vi "Icai 105 - Simultry4.vi"() -> ()   [LabVIEW 2010]
uses:
  <vilib>/Utility/error.llb/DialogType.ctl
  <vilib>/DAQmx/write.llb/DAQmx Write (Analog DBL 1Chan 1Samp).vi
  <vilib>/DAQmx/write.llb/DAQmx Write (Analog Wfm 1Chan NSamp).vi
  <vilib>/DAQmx/create/channels.llb/DAQmx Create Channel (AO-Voltage-Basic).vi
  <vilib>/daqmx/miscellaneous.llb/DAQmx Fill In Error Info.vi
  <vilib>/Waveform/WDTOps.llb/WDT Append Waveforms DBL.vi
  <vilib>/measure/NI_MABase.lvlib
  Program Files/National Instruments/LabVIEW 2010/resource/objmgr/daqmx.rc
panel:
  in  "Rising Logic Output Chan":tag="Dev1/ao2"
  in  "Modulation Duration samples / 2":i32=150000
  out "Multiplier to arrive at Modulation # of samples":dbl=297.555285
  in  "Samples (1Ms/s)":i32=700000
  out "Name":refnum<k21>
  out "number of samples written per channel":u32
  out "min value":dbl
  in  "Falling Logic Output Chan":tag="Dev1/ao1"
  in  "FM Waveform Channel":tag="Dev1/ao3"
  out "error out":errorcluster caption="error out (DAQ)"
  out "Mod":dbl=118572.0
  out "Numeric 2":dbl=3900000.0 format="%#_7g"
  out "Numeric":dbl=3900000.0 format="%#_7g"
  in  "CAI/ICAI":bool=TRUE
  in  "Pre-Trig Samples":ext=500.0 format="%.2f"
  out "?":dbl=579698.7113293351 format="%#_6f"
  in  "Fs":dbl=1000000.0
  out "#s":dbl=39524.02451426849
  in  "Time int":i32=30000
  in  "Sensitivity":u16(ring)=14 items=["2 nV/fA", "5 nV/fA", "10 nV/fA", "20 nV/fA", "50 nV/fA", "100 nV/fA", "200 nV/fA", "500 nV/fA", "1 uV/pA", "2 uV/pA", "5 uV/pA", "10 uV/pA", "20 uV/pA", "50 uV/pA", "100 uV/pA", "200 uV/pA", "500 uV/pA", "1 mV/nA", "2 mV/nA", "5 mV/nA", "10 mV/nA", "20 mV/nA", "50 mV/nA", "100 mV/nA", "200 mV/nA", "500 mV/nA", "1 V/uA"]
  in  "Detection Bandwidth":u16(ring)=7 items=["10 us/ 25 kHz", "30 us /8.33 kHz", "100 us/ 2.50 kHz", "300 us/ 833 Hz", "1 ms /250 Hz", "3 ms /83.3 Hz", "10 ms/ 25 Hz", "30 ms/ 8.33 Hz", "100 ms/ 2.50 Hz", "300 ms/ 0.833 Hz ", "1 s/ 0.250 Hz", "3 s/ 0.0833 Hz", "10 s/0.025 Hz"]
  in  "SR 830 GPIB Address":i32=8
  in  "Freq 2":dbl=2490.2 format="%_7g"
  out "Iterat #":dbl=10.0
  in  "Iteration":dbl=17.0
  in  "stop 2":bool
  in  "pulse":bool=TRUE
  in  "Start":ext=0.05
  out "?":waveform(dbl)[](graph)
  in  "amplitude 2":dbl=0.2 format="%0.2p"
  in  "?":T1(ring)
  in  "phase 2":dbl format="%.2p"
  in  "Offset 2":dbl=-0.0 format="%#_6p"
  in  "frequency 4":dbl=100.0 format="%0.2p"
  in  "sampling info 4":cluster{"Fs":dbl, "#s":dbl}={"Fs"=1000000.0, "#s"=2500.0} {"Fs" format="%.2p"}
  in  "?":T1(ring)=enum."Triangle Wave"
  in  "offset 4":dbl=-1.0 format="%0.2p"
  in  "phase 4":dbl=90.0 format="%.2p"
  in  "amplitude 4":dbl=1.0 format="%0.2p"
  in  "frequency 1":dbl=100.0 format="%0.2p"
  in  "amplitude 1":dbl=1.0 format="%0.2p"
  in  "sampling info 1":cluster{"Fs":dbl, "#s":dbl}={"Fs"=1000000.0, "#s"=2500.0} {"Fs" format="%.2p"}
  in  "?":T1(ring)=enum."Triangle Wave"
  in  "phase 1":dbl=-90.0 format="%.2p"
  in  "Offset 1":dbl format="%#_6p"
  in  "iterat":dbl=1.0
  out "CW":dbl=123571.0
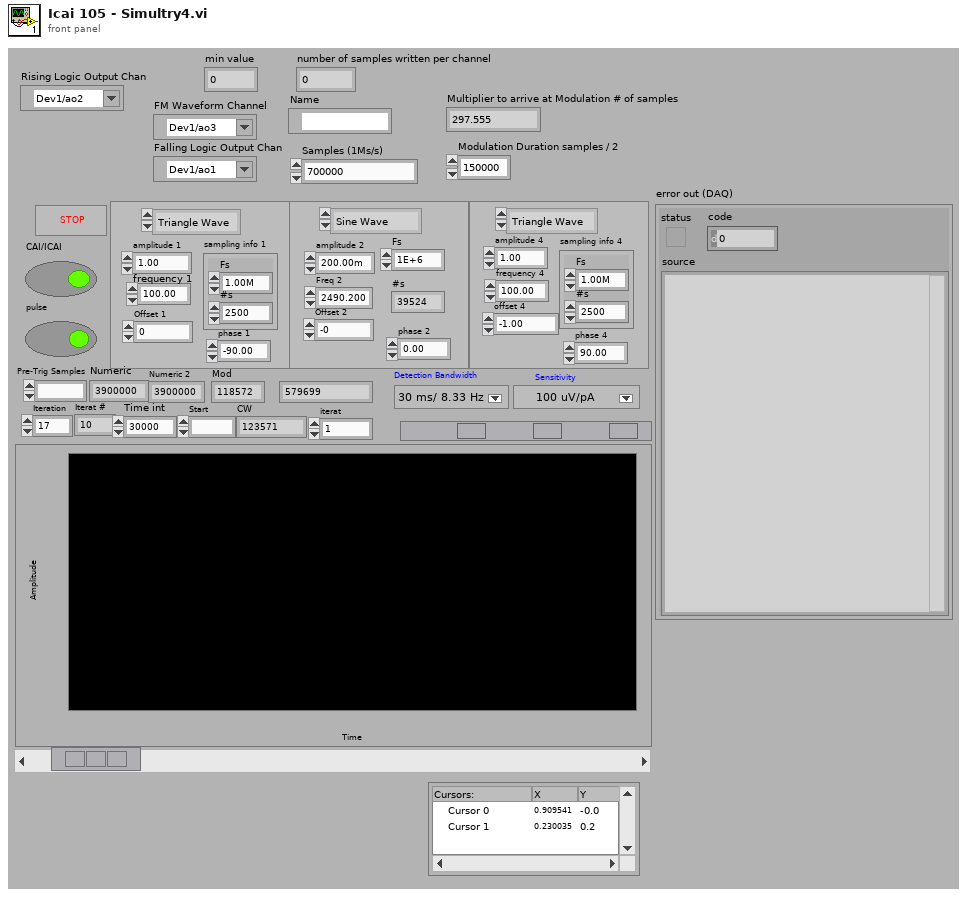
[diagram p1: front panel]
types:
  T1 = enum16{"Sine Wave", "Triangle Wave", "Square Wave", "Sawtooth Wave"}
  T2 = typedef "DialogType.ctl" = u16
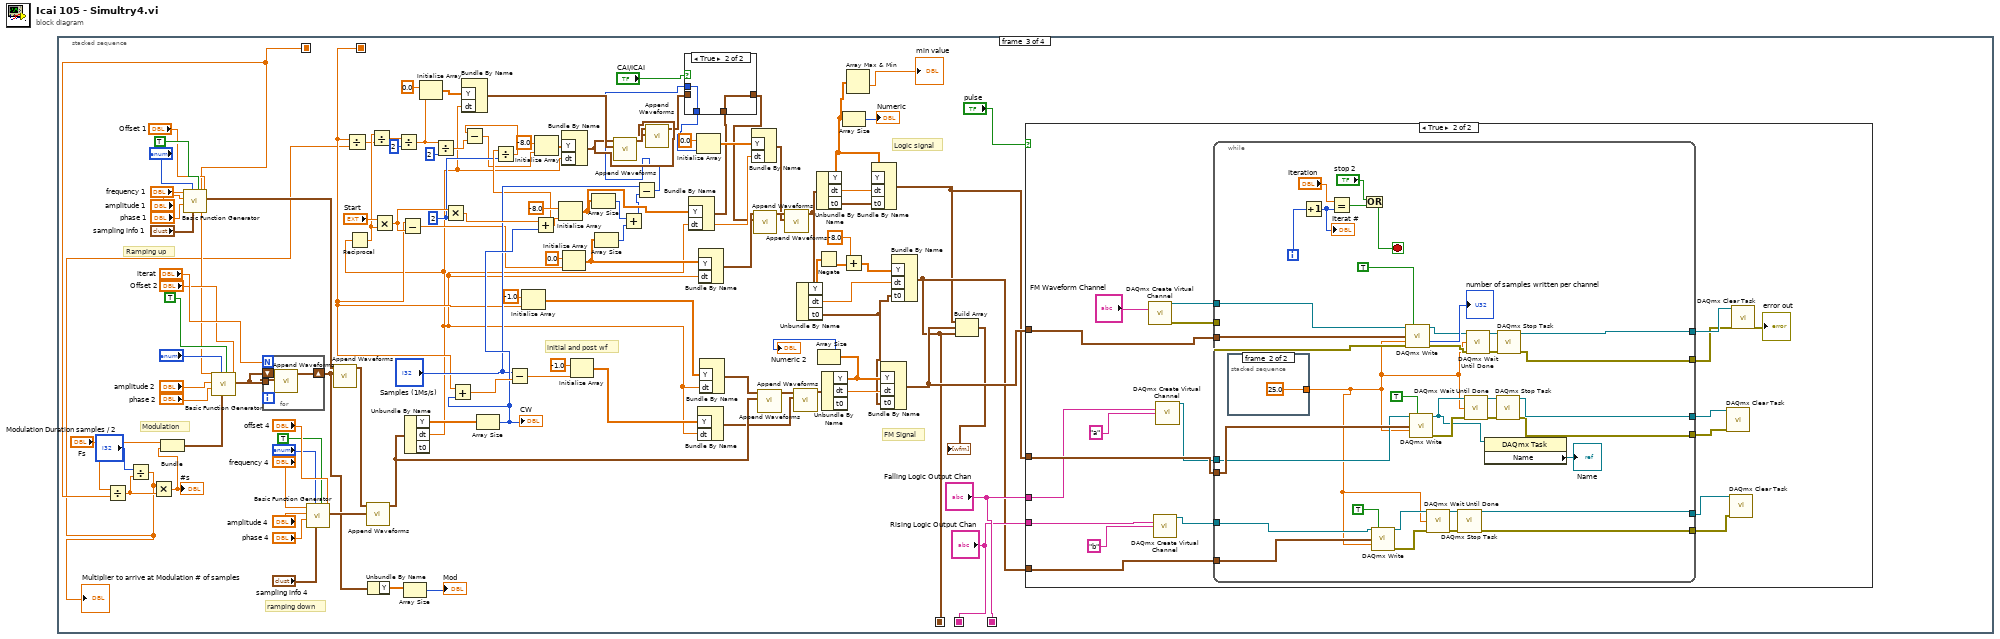
[diagram p0: block diagram]
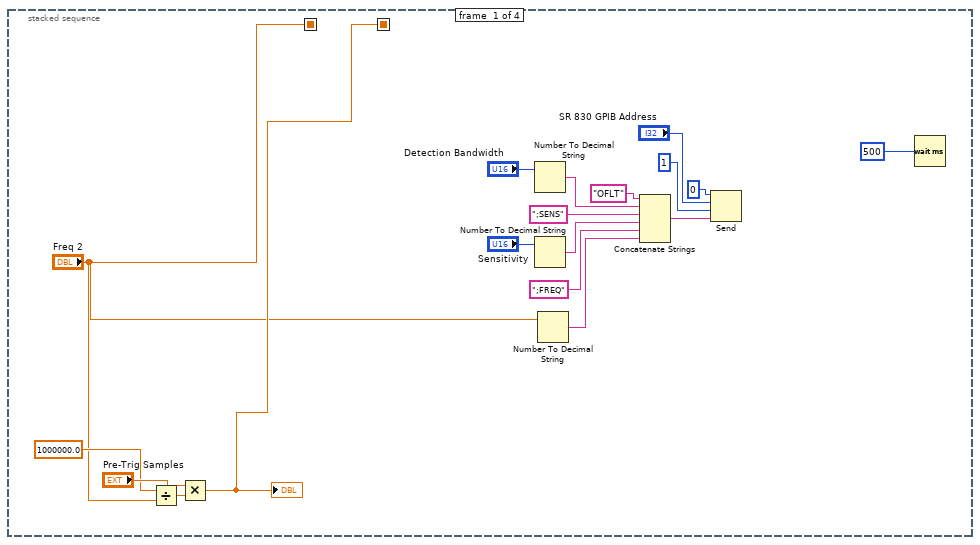
[diagram p2: hidden frame]
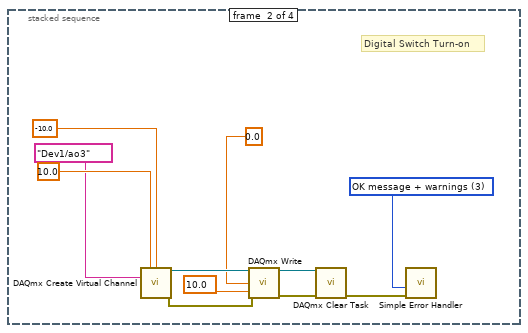
[diagram p3: hidden frame]
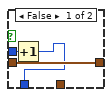
[diagram p4: hidden frame]
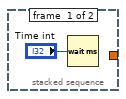
[diagram p6: hidden frame]
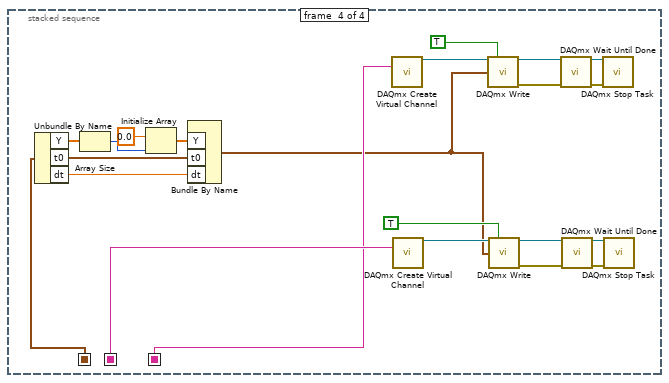
[diagram p7: hidden frame]
diagram:
  n1 = stacked-sequence {
    seq-local: ["Freq 2" _ _ _] -> [_ _ w84 _]
    seq-local: [w4 _ _ _] -> [_ _ w71 _]
    seq-local: [_ _ "Falling Logic Output Chan" _] -> [_ _ _ w209]
    seq-local: [_ _ "Rising Logic Output Chan" _] -> [_ _ _ w210]
    seq-local: [_ _ w32 _] -> [_ _ _ w224]
    frame #0 {
      n2 = Divide(x=1000000.0 ("Fs 2"), y="Freq 2") -> (x/y=w7:dbl)
      n3 = Multiply(x="Pre-Trig Samples", y=w7) -> (x*y=w4:ext)
      "?" <- w4
      n4 = Number To Decimal String(number="Detection Bandwidth") -> (decimal integer string=w17:string)  [unwired: 1 out]
      n5 = Number To Decimal String(number="Sensitivity") -> (decimal integer string=w15:string)  [unwired: 1 out]
      n6 = Number To Decimal String(number="Freq 2") -> (decimal integer string=w2:string)  [unwired: 1 out]
      n7 = Concatenate Strings("OFLT", w17, ";SENS", w15, ";FREQ" ("string"), w2) -> (w14:string)
      n8 = Send(0:0 ("bus"), 2:"SR 830 GPIB Address", 3:i16 1 ("mode"), 5:w14) -> ()  [unwired: 1 in, 3 out]
      n9 = Wait (ms)(milliseconds to wait=500) -> ()  [unwired: 1 out]
    }
    frame #1 {
      w22 = T2 3 items=["no dialog", "OK message", "continue or stop message", "OK message + warnings", "continue/stop + warnings"] ("type of dialog (OK msg:1)")
      # "Digital Switch Turn-on"
      n10 = call-poly <vilib>:"DAQmx Create Virtual Channel.vi"("maximum value"=10.0 ("Maximum Value"), "minimum value"=-10.0 ("Minimum Value"), "physical channels"=tag "Dev1/ao3" ("Physical Channel")) -> ("task out"=w25:refnum<k21>, "error out"=w26:errorcluster)  [unwired: 6 in, 5 out]
      n11 = call-poly <vilib>:"DAQmx Write.vi"("task/channels in"=w25, "data"=0.0 ("Voltage Output"), "timeout"=10.0, "error in"=w26) -> ("task out"=w20:refnum<k21>, "error out"=w21:errorcluster)  [unwired: 1 in, 9 out]
      n12 = call <vilib>:"DAQmx Clear Task.vi"("task in"=w20, "error in"=w21) -> ("error out"=w19:errorcluster)  [unwired: 13 out]
      n13 = call <vilib>:"Simple Error Handler.vi"("type of dialog (OK msg:1)"=w22, "error in (no error)"=w19) -> ()  [unwired: 8 out]
    }
    frame #2 {
      w79 = 2
      # "initial and post wf"
      # "FM Signal"
      # "Logic signal"
      # "Ramping up"
      # "ramping down"
      # "Modulation"
      n14 = Divide(x="Fs", y=w84) -> (x/y=w45:dbl)
      n15 = Divide(x="Modulation Duration samples / 2", y=w45) -> (x/y=w44:dbl)
      "Multiplier to arrive at Modulation # of samples" <- w44
      n16 = Multiply(x=w44, y=w45) -> (x*y=w47:dbl)
      "#s" <- w47
      n17 = Bundle("Fs"="Fs", w47) -> (w82:cluster{"Fs":dbl, dbl})  [unwired: 1 out]
      n18 = call <vilib>:"Basic Function Generator.vi"("offset"="Offset 1", "reset signal"=TRUE, "sampling info"="sampling info 1", "signal type"="?", "phase"="phase 1", "amplitude"="amplitude 1", "frequency"="frequency 1") -> ("signal out"=w120:waveform(dbl))  [unwired: 2 in, 2 out]
      n19 = call <vilib>:"Basic Function Generator.vi"("offset"="Offset 2", "reset signal"=TRUE, "sampling info"=w82, "signal type"="?", "phase"="phase 2", "amplitude"="amplitude 2", "frequency"=w84) -> ("signal out"=w85:waveform(dbl))  [unwired: 2 in, 2 out]
      n20 = for {
        N: "iterat" -> [_]
        shift-right: [w207] -> w50
        shift-left: w85 -> [w205]
        tunnel: w85 -> [w206]
        n21 = call-poly <vilib>:"Append Waveforms.vi"("waveform B"=w206, "waveform A"=w205) -> ("waveform out"=w207:waveform(dbl))  [unwired: 1 in, 8 out]
      }
      n22 = call <vilib>:"Basic Function Generator.vi"("offset"="offset 4", "reset signal"=TRUE, "sampling info"="sampling info 4", "signal type"="?", "phase"="phase 4", "amplitude"="amplitude 4", "frequency"="frequency 4") -> ("signal out"=w125:waveform(dbl))  [unwired: 2 in, 2 out]
      n23 = call-poly <vilib>:"Append Waveforms.vi"("waveform B"=w50, "waveform A"=w120) -> ("waveform out"=w119:waveform(dbl))  [unwired: 1 in, 8 out]
      n24 = Divide(x=w71, y=w44) -> (x/y=w72:ext)
      n25 = call-poly <vilib>:"Append Waveforms.vi"("waveform B"=w125, "waveform A"=w119) -> ("waveform out"=w118:waveform(dbl))  [unwired: 1 in, 8 out]
      n26 = Unbundle By Name(w50) -> ("Y"=w51:dbl[])
      n27 = Array Size(array=w51) -> (size(s)=→"Mod":i32)
      n28 = Unbundle By Name(w118) -> ("Y"=w121:dbl[], "dt"=w63:dbl)  [unwired: 1 out]
      n29 = Reciprocal(x=w63) -> (1/x=w73:dbl)
      n30 = Divide(x=w73, y=w72) -> (x/y=w69:ext)
      n31 = Multiply(x="Start", y=w73) -> (x*y=w95:ext)
      n32 = Divide(x=w69, y=2) -> (x/y=w66:ext)
      n33 = Subtract(x=w71, y=w95) -> (x-y=w96:ext)
      n34 = Initialize Array(0.0 ("Trigger down"), w66) -> (w76:dbl[])
      n35 = Divide(x=w66, y=2) -> (x/y=w64:ext)
      n36 = Multiply(x=w95, y=w79) -> (x*y=w103:ext)
      n37 = Bundle By Name("Y"=w76, "dt"=w63) -> (w75:waveform(dbl))  [unwired: 1 out]
      n38 = Array Size(array=w121) -> (size(s)=w102:i32)
      "CW" <- w102
      n39 = Add(x=w71, y=w102) -> (x+y=w107:ext)
      n40 = Subtract(x="Samples (1Ms/s)", y=w107) -> (x-y=w106:ext)
      n41 = Initialize Array(-1.0 ("DC level"), w71) -> (w109:dbl[])
      n42 = Add(x=w103, y=w102) -> (x+y=w80:ext)
      n43 = Divide(x=w80, y=w79) -> (x/y=w68:ext)
      n44 = Subtract(x=w68, y=w64) -> (x-y=w67:ext)
      n45 = Initialize Array(-8.0 ("Trigger up"), w67) -> (w78:dbl[])
      n46 = Initialize Array(-8.0 ("Trigger up"), w80) -> (w93:dbl[])
      n47 = Bundle By Name("Y"=w78, "dt"=w63) -> (w62:waveform(dbl))  [unwired: 1 out]
      n48 = Initialize Array(0.0 ("Trigger down"), w96) -> (w94:dbl[])
      n49 = Initialize Array(-1.0 ("DC level"), w106) -> (w105:dbl[])
      n50 = Array Size(array=w93) -> (size(s)=w91:i32)
      n51 = Array Size(array=w94) -> (size(s)=w92:i32)
      n52 = call-poly <vilib>:"Append Waveforms.vi"("waveform B"=w75, "waveform A"=w62) -> ("waveform out"=w74:waveform(dbl))  [unwired: 1 in, 8 out]
      n53 = Add(x=w91, y=w92) -> (x+y=w90:i32)
      n54 = Subtract(x="Samples (1Ms/s)", y=w90) -> (x-y=w54:i32)
      n55 = call-poly <vilib>:"Append Waveforms.vi"("waveform B"=w62, "waveform A"=w74) -> ("waveform out"=w61:waveform(dbl))  [unwired: 1 in, 8 out]
      n56 = Bundle By Name("Y"=w93, "dt"=w63) -> (w59:waveform(dbl))  [unwired: 1 out]
      n57 = case shown="True" "CAI/ICAI" {
        tunnel: w61 -> [w144 _]
        tunnel: [w144 w146] -> w60
        tunnel: w59 -> [_ w146]
        tunnel: w54 -> [w143 w145]
        tunnel: [w142 w145] -> w53
        frame False {
          n58 = Increment(x=w143) -> (x+1=w142:i32)
        }
        frame True {
        }
      }
      n59 = Initialize Array(0.0 ("Trigger down"), w53) -> (w99:dbl[])
      n60 = Bundle By Name("Y"=w105, "dt"=w63) -> (w104:waveform(dbl))  [unwired: 1 out]
      n61 = Bundle By Name("Y"=w94, "dt"=w63) -> (w98:waveform(dbl))  [unwired: 1 out]
      n62 = Bundle By Name("Y"=w109, "dt"=w63) -> (w123:waveform(dbl))  [unwired: 1 out]
      n63 = Bundle By Name("Y"=w99, "dt"=w63) -> (w97:waveform(dbl))  [unwired: 1 out]
      n64 = call-poly <vilib>:"Append Waveforms.vi"("waveform B"=w60, "waveform A"=w98) -> ("waveform out"=w115:waveform(dbl))  [unwired: 1 in, 8 out]
      n65 = call-poly <vilib>:"Append Waveforms.vi"("waveform B"=w118, "waveform A"=w123) -> ("waveform out"=w124:waveform(dbl))  [unwired: 1 in, 8 out]
      n66 = call-poly <vilib>:"Append Waveforms.vi"("waveform B"=w97, "waveform A"=w115) -> ("waveform out"=w43:waveform(dbl))  [unwired: 1 in, 8 out]
      n67 = call-poly <vilib>:"Append Waveforms.vi"("waveform B"=w104, "waveform A"=w124) -> ("waveform out"=w112:waveform(dbl))  [unwired: 1 in, 8 out]
      n68 = Unbundle By Name(w43) -> ("Y"=w42:dbl[], "dt"=w37:dbl, "t0"=w38:timestamp)
      n69 = Unbundle By Name(w43) -> ("Y"=w49:dbl[], "dt"=w113:dbl, "t0"=w39:timestamp)
      n70 = Negate(x=w42) -> (-x=w40:dbl[])
      n71 = Unbundle By Name(w112) -> ("Y"=w55:dbl[], "dt"=w111:dbl)  [unwired: 1 out]
      n72 = Array Size(array=w55) -> (size(s)=→"Numeric 2":i32)
      n73 = Add(x=-8.0, y=w40) -> (x+y=w36:dbl[])
      n74 = Array Size(array=w49) -> (size(s)=→"Numeric":i32)
      n75 = Array Max & Min(array=w49) -> (min value=→"min value":dbl)  [unwired: 3 out]
      n76 = Bundle By Name("Y"=w49, "dt"=w113, "t0"=w39) -> (w31:waveform(dbl))  [unwired: 1 out]
      n77 = Bundle By Name("Y"=w55, "dt"=w111, "t0"=w38) -> (w48:waveform(dbl))  [unwired: 1 out]
      n78 = Bundle By Name("Y"=w36, "dt"=w37, "t0"=w38) -> (w32:waveform(dbl))  [unwired: 1 out]
      n79 = Build Array(w31, w48, w32) -> (→"?":waveform(dbl)[])
      n80 = case shown="True" "pulse" {
        tunnel: w48 -> [_ w165]
        tunnel: w31 -> [_ w161]
        tunnel: w32 -> [_ w149]
        tunnel: "Falling Logic Output Chan" -> [_ w147]
        tunnel: "Rising Logic Output Chan" -> [_ w148]
        frame False {
        }
        frame True {
          n81 = call-poly <vilib>:"DAQmx Create Virtual Channel.vi"("physical channels"="FM Waveform Channel") -> ("task out"=w163:refnum<k21>, "error out"=w162:errorcluster)  [unwired: 13 in]
          n82 = call-poly <vilib>:"DAQmx Create Virtual Channel.vi"("physical channels"=w148, "name to assign"="b") -> ("task out"=w152:refnum<k21>)  [unwired: 12 in, 1 out]
          n83 = call-poly <vilib>:"DAQmx Create Virtual Channel.vi"("physical channels"=w147, "name to assign"="a") -> ("task out"=w159:refnum<k21>)  [unwired: 12 in, 1 out]
          n84 = while {
            tunnel: w165 -> [w190]
            tunnel: w163 -> [w184]
            tunnel: w162 -> [w183]
            tunnel: w161 -> [w187]
            tunnel: w159 -> [w182]
            tunnel: [w179] -> w158
            tunnel: [w178] -> w157
            tunnel: [w177] -> w156
            tunnel: [w176] -> w155
            tunnel: w152 -> [w168]
            tunnel: [w170] -> w151
            tunnel: [w169] -> w150
            tunnel: w149 -> [w167]
            i -> [w199]
            stop <- w200 stop-if-true
            n85 = stacked-sequence {
              tunnel: [_ 25.0 ("timeout (s)")] -> w166
              frame #0 {
                n86 = Wait (ms)(milliseconds to wait="Time int") -> ()  [unwired: 1 out]
              }
              frame #1 {
              }
            }
            n87 = Increment(x=w199) -> (x+1=w197:i32)
            "Iterat #" <- w197
            n88 = Equal?(x="Iteration", y=w197) -> (x = y?=w202:bool)
            n89 = Or(x="stop 2", y=w202) -> (x .or. y?=w200:bool)
            n90 = call-poly <vilib>:"DAQmx Write.vi"("task/channels in"=w168, "auto start"=TRUE, "data"=w167, "timeout"=w166) -> ("task out"=w171:refnum<k21>, "error out"=w174:errorcluster)  [unwired: 9 in, 1 out]
            n91 = call-poly <vilib>:"DAQmx Write.vi"("task/channels in"=w184, "auto start"=TRUE, "data"=w190, "timeout"=w166, "error in"=w183) -> ("task out"=w192:refnum<k21>, "number of samples written per channel"=→"number of samples written per channel":u32, "error out"=w191:errorcluster)  [unwired: 8 in]
            n92 = call-poly <vilib>:"DAQmx Write.vi"("task/channels in"=w182, "auto start"=TRUE, "data"=w187, "timeout"=w166) -> ("task out"=w181:refnum<k21>, "error out"=w188:errorcluster)  [unwired: 9 in, 1 out]
            n93 = call <vilib>:"DAQmx Wait Until Done.vi"("task/channels in"=w171, "timeout (sec)"=w166, "error in"=w174) -> ("task out"=w173:refnum<k21>, "error out"=w175:errorcluster)  [unwired: 11 in]
            n94 = call <vilib>:"DAQmx Stop Task.vi"("task/channels in"=w173, "error in"=w175) -> ("task out"=w170:refnum<k21>, "error out"=w169:errorcluster)  [unwired: 12 in]
            n95 = call <vilib>:"DAQmx Wait Until Done.vi"("task/channels in"=w181, "timeout (sec)"=w166, "error in"=w188) -> ("task out"=w186:refnum<k21>, "error out"=w189:errorcluster)  [unwired: 11 in]
            n96 = call <vilib>:"DAQmx Wait Until Done.vi"("task/channels in"=w192, "timeout (sec)"=w166, "error in"=w191) -> ("task out"=w196:refnum<k21>, "error out"=w195:errorcluster)  [unwired: 11 in]
            n97 = property class="DAQmx Task"(reference=w181) -> ("Name"=→"Name":refnum<k21>)  [unwired: 1 in, 2 out]
            n98 = call <vilib>:"DAQmx Stop Task.vi"("task/channels in"=w186, "error in"=w189) -> ("task out"=w179:refnum<k21>, "error out"=w178:errorcluster)  [unwired: 12 in]
            n99 = call <vilib>:"DAQmx Stop Task.vi"("task/channels in"=w196, "error in"=w195) -> ("task out"=w177:refnum<k21>, "error out"=w176:errorcluster)  [unwired: 12 in]
          }
          n100 = call <vilib>:"DAQmx Clear Task.vi"("task in"=w158, "error in"=w157) -> ()  [unwired: 13 in, 1 out]
          n101 = call <vilib>:"DAQmx Clear Task.vi"("task in"=w151, "error in"=w150) -> ()  [unwired: 13 in, 1 out]
          n102 = call <vilib>:"DAQmx Clear Task.vi"("task in"=w156, "error in"=w155) -> ("error out"=→"error out":errorcluster)  [unwired: 13 in]
        }
      }
    }
    frame #3 {
      n103 = Unbundle By Name(w224) -> ("Y"=w221:dbl[], "t0"=w223:timestamp, "dt"=w222:dbl)
      n104 = Array Size(array=w221) -> (size(s)=w220:i32)
      n105 = Initialize Array(0.0 ("element"), w220) -> (w218:dbl[])
      n106 = Bundle By Name("Y"=w218, "t0"=w223, "dt"=w222) -> (w208:waveform(dbl))  [unwired: 1 in]
      n107 = call-poly <vilib>:"DAQmx Create Virtual Channel.vi"("physical channels"=w209) -> ("task out"=w217:refnum<k21>)  [unwired: 13 in, 1 out]
      n108 = call-poly <vilib>:"DAQmx Create Virtual Channel.vi"("physical channels"=w210) -> ("task out"=w211:refnum<k21>)  [unwired: 13 in, 1 out]
      n109 = call-poly <vilib>:"DAQmx Write.vi"("task/channels in"=w217, "auto start"=TRUE, "data"=w208) -> ("task out"=w225:refnum<k21>, "error out"=w228:errorcluster)  [unwired: 10 in, 1 out]
      n110 = call-poly <vilib>:"DAQmx Write.vi"("task/channels in"=w211, "auto start"=TRUE, "data"=w208) -> ("task out"=w212:refnum<k21>, "error out"=w215:errorcluster)  [unwired: 10 in, 1 out]
      n111 = call <vilib>:"DAQmx Wait Until Done.vi"("task/channels in"=w225, "error in"=w228) -> ("task out"=w227:refnum<k21>, "error out"=w229:errorcluster)  [unwired: 12 in]
      n112 = call <vilib>:"DAQmx Wait Until Done.vi"("task/channels in"=w212, "error in"=w215) -> ("task out"=w214:refnum<k21>, "error out"=w216:errorcluster)  [unwired: 12 in]
      n113 = call <vilib>:"DAQmx Stop Task.vi"("task/channels in"=w227, "error in"=w229) -> ()  [unwired: 12 in, 2 out]
      n114 = call <vilib>:"DAQmx Stop Task.vi"("task/channels in"=w214, "error in"=w216) -> ()  [unwired: 12 in, 2 out]
    }
  }
